vi "Close.vi"(8 "error in (no error)":errorcluster, 11 "NetworkStreamReader in":refnum<class "NetworkStreamReader.lvclass">) -> (0 "error out":errorcluster, 3 "NetworkStreamReader out":refnum<class "NetworkStreamReader.lvclass">)   [LabVIEW 2011, in "NetworkStreamReader.lvclass"]
doc: "This VI closes references internal to the NetworkStreamReader object. This allows memory to be cleaned up effectively."
uses:
  NetworkStreamReader.lvclass
  NetworkStreamReader.lvclass/NetworkStreamReader.ctl
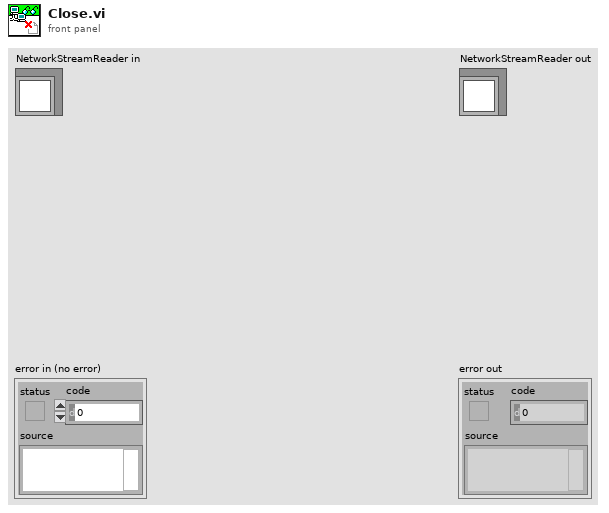
[diagram p1: front panel]
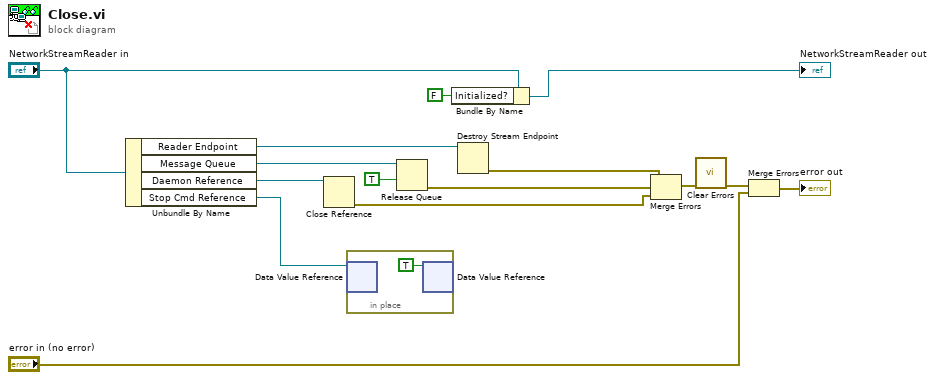
[diagram p0: block diagram]
diagram:
  n1 = Unbundle By Name("NetworkStreamReader in") -> ("Reader Endpoint"=w10:refnum<k21>, "Message Queue"=w14:refnum<queue>, "Daemon Reference"=w15:refnum<vi>, "Stop Cmd Reference"=w12:refnum<data-value>)
  n2 = Close Reference(reference=w15) -> (error out=w8:errorcluster)  [unwired: 1 in]
  n3 = in-place {
    n4 = in-place-dvr #1(w12) -> ()  [unwired: 2 out]
    n5 = in-place-dvr #1(TRUE ("data value")) -> ()  [unwired: 2 out]
  }
  n6 = Release Queue(queue=w14, force destroy? (F)=TRUE) -> (error out=w9:errorcluster)  [unwired: 1 in, 2 out]
  n7 = Bundle By Name(cluster="NetworkStreamReader in", "Initialized?"=FALSE) -> (→"NetworkStreamReader out":refnum<class "NetworkStreamReader.lvclass">)
  n8 = Destroy Stream Endpoint(11:w10) -> (0:w11:errorcluster)  [unwired: 1 in]
  n9 = Merge Errors(w11, w9, w8) -> (w7:errorcluster)
  n10 = call <vilib>:"Clear Errors.vi"("error in (no error)"=w7) -> ("error out"=w6:errorcluster)  [unwired: 6 in]
  n11 = Merge Errors(w6, "error in (no error)") -> (→"error out":errorcluster)
